vi "ReadConfig.vi"(8 "error in (no error)":errorcluster, 11 "GRMActor in":refnum<class "CameraController.lvclass">) -> (0 "error out":errorcluster, 3 "GRMActor out":refnum<class "CameraController.lvclass">)   [LabVIEW 2020, in "CameraController.lvlib" / "CameraController.lvclass"]
uses:
  CameraController.lvclass
  CameraController.lvclass/CameraController.ctl
  Model/Hardware Abstraction Layer/Component/GenericActor/GenericActor/GenericController.lvclass
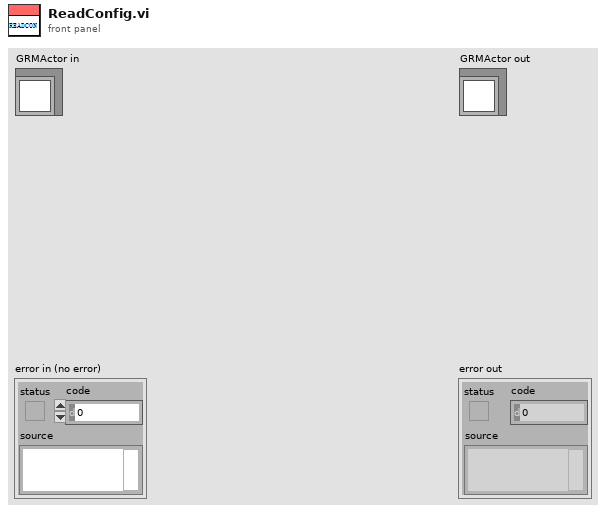
[diagram p1: front panel]
types:
  T1 = typedef "NI_LVConfig.lvlib/Config Data RefNum.ctl" = refnum<k1>
  T2 = cluster{"Values[0]":dbl, "Values[1]":dbl, "Values[2]":dbl, "Values[3]":dbl}
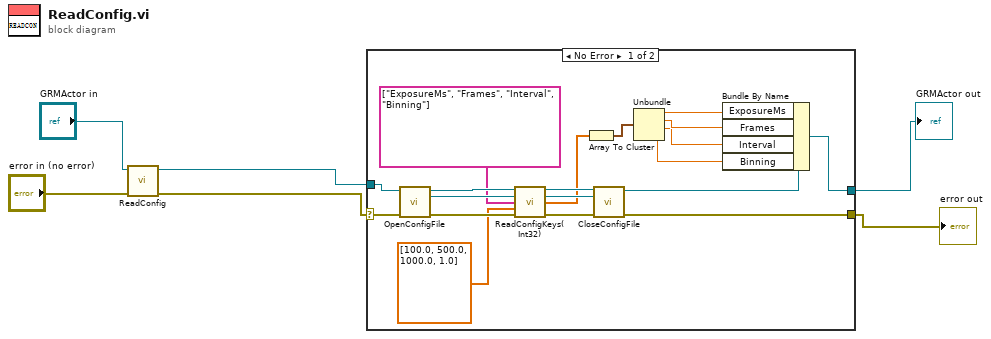
[diagram p0: block diagram]
diagram:
  n1 = call-parent "ReadConfig.vi"("error in (no error)"="error in (no error)", "GRMActor in"="GRMActor in") -> ("error out"=w3:errorcluster, "GRMActor out"=w4:refnum<class "CameraController.lvclass">)  [unwired: 8 in]
  n2 = case shown="No Error" w3 {
    selector: w3 -> [w25 w26]
    tunnel: [w18 w26] -> w1
    tunnel: [w12 w27] -> w2
    tunnel: w4 -> [w24 w27]
    frame No Error {
      n3 = call-dynamic "OpenConfigFile.vi"("error in (no error)"=w25, "GRMActor in"=w24) -> ("error out"=w23:errorcluster, "refnum"=w19:T1, "GRMActor out"=w21:refnum<class "CameraController.lvclass">)  [unwired: 7 in]
      n4 = call-dynamic "ReadConfigKeys(Int32).vi"("GRMActor in"=w21, "Config Refnum"=w19, "Keys"=string[] ["ExposureMs", "Frames", "Interval", "Binning"] ("Values"), "Default"=dbl[] [100.0, 500.0, 1000.0, 1.0], "error in (no error)"=w23) -> ("GRMActor out"=w17:refnum<class "CameraController.lvclass">, "Config Refnum dup"=w16:T1, "Values"=w15:dbl[], "error out"=w22:errorcluster)  [unwired: 7 in]
      n5 = Array To Cluster(array=w15) -> (cluster=w20:T2)
      n6 = call-dynamic "CloseConfigFile.vi"("error in (no error)"=w22, "refnum"=w16, "GRMActor in"=w17) -> ("error out"=w18:errorcluster, "GRMActor out"=w13:refnum<class "CameraController.lvclass">)  [unwired: 7 in]
      n7 = Unbundle(w20) -> ("Values[0]"=w10:dbl, "Values[1]"=w9:dbl, "Values[2]"=w8:dbl, "Values[3]"=w7:dbl)
      n8 = Bundle By Name(cluster=w13, "ExposureMs"=w10, "Frames"=w9, "Interval"=w8, "Binning"=w7) -> (w12:refnum<class "CameraController.lvclass">)
    }
    frame Error {
    }
  }
  "error out" <- w1
  "GRMActor out" <- w2
